vi "Main.vi"() -> ()   [LabVIEW 2021]
uses:
  Sub VIs/State Estimator/Measurements.ctl
  Sub VIs/IMU/IMU Data.ctl
  Sub VIs/Steering Motor Encoder/Steering Motor Encoder Data.ctl
  Sub VIs/GNSS/GNSS Data.ctl
  Sub VIs/State Estimator/State Estimate.ctl
  Sub VIs/Logging/Controller Data.ctl
  Sub VIs/Drive Motor/Drive Motor Data.ctl
  Sub VIs/Steering Motor/Steering Motor Data.ctl
  <vilib>/Utility/RT CPU Load.ctl
  Sub VIs/Trajectory Control/Trajectory_Control.ctl
  Sub VIs/Logging/Log Level.ctl
  <vilib>/Platform/TimedLoop/XDataNode/timing_clust.ctl
  <vilib>/Platform/TimedLoop/XDataNode/nitl_modes.ctl
  <vilib>/Platform/TimedLoop/XDataNode/wakeup.ctl
  <vilib>/platform/TimedLoop/XDataNode/XDataNode.xnode
  <vilib>/Platform/TimedLoop/XDataNode/XDNodeRunTimeDep.lvlib
  <vilib>/NI_Real-Time Target Support.lvlib
panel:
  out "XY trajectory (0 is bikeposition)":T1(graph)
  out "Y-Offset":dbl
  out "X-Offset":dbl
  out "Trajectory (Debug)":T2
  in  "Reset and Init trajectory":bool
  out "CPU loads":T3[](array[typedef]) {"ISR (%)" format="%#.2f"; "Idle (%)" format="%#.2f"; "Background (%)" format="%#.2f"; "Normal (%)" format="%#.2f"; "Above Normal (%)" format="%#.2f"; "High (%)" format="%#.2g"; "Timed Structures (%)" format="%#.2g"; "Time Critical (%)" format="%#.2g"; "Total (%)" format="%#.2g"}
  in  "Drive Motor Angular Speed (rad/s)":dbl
  out "Motor Controllers (Debug)":T4
  in  "Enable Steering Motor":bool
  out "Steering Motor Enabled":bool
  out "State Estimate (Debug)":T7 {"Y (m)" format="%#_10g"; "X (m)" format="%#_10g"}
  out "Measurements (Debug)":T8 {"GNSS Data"."Longitude (deg)" format="%#.10g"; "GNSS Data"."Latitude (deg)" format="%#.10g"; "GNSS Data"."Longitude (rad)" format="%#_10g"; "GNSS Data"."Latitude (rad)" format="%#_10g"}
  out "Abort":bool
  in  "Reset Steering Motor Encoder":bool
  in  "Stop Button":bool
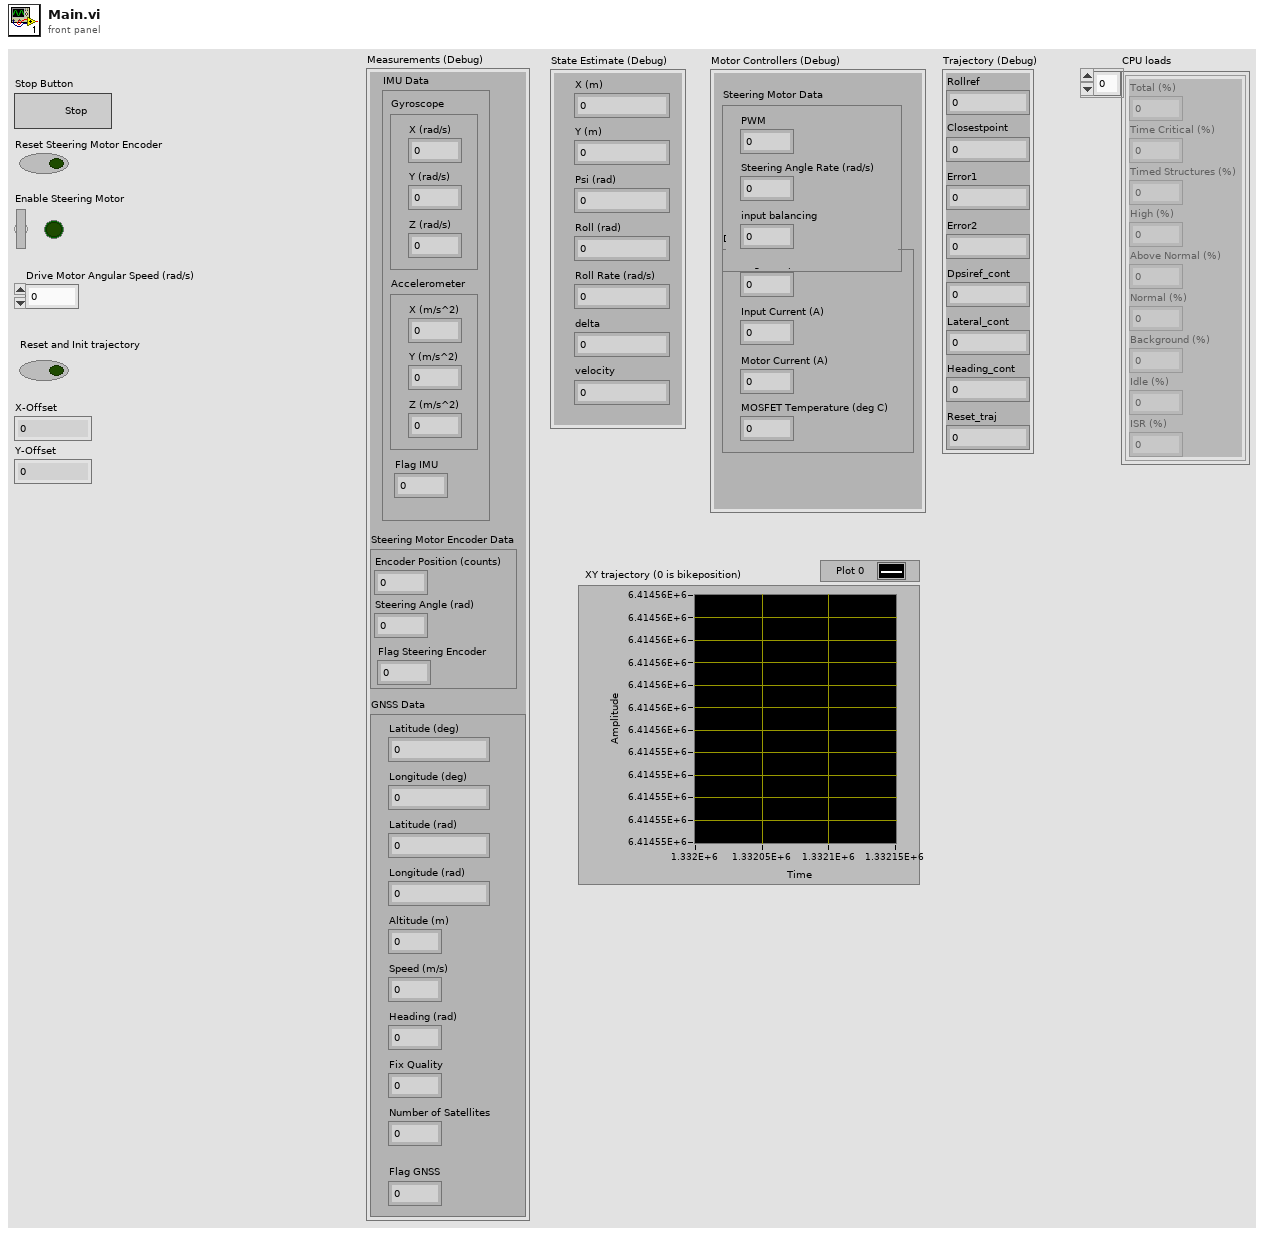
[diagram p1: front panel]
types:
  T1 = cluster{"Trajectory(X/Y/PSI)":dbl[], "Trajectory(X/Y/PSI)":dbl[]}
  T2 = typedef "Trajectory_Control.ctl" = cluster{"Rollref":dbl, "Closestpoint":dbl, "Error1":dbl, "Error2":dbl, "Dpsiref_cont":dbl, "Lateral_cont":dbl, "Heading_cont":dbl, "Reset_traj":dbl}
  T3 = typedef "NI_Real-Time Target Support.lvlib/RT CPU Load.ctl" = cluster{"Total (%)":dbl, "Time Critical (%)":dbl, "Timed Structures (%)":dbl, "High (%)":dbl, "Above Normal (%)":dbl, "Normal (%)":dbl, "Background (%)":dbl, "Idle (%)":dbl, "ISR (%)":dbl}
  T4 = typedef "Controller Data.ctl" = cluster{"Drive Motor Data":T5, "Steering Motor Data":T6}
  T5 = typedef "Drive Motor Data.ctl" = cluster{"Angular Speed (rad/s)":dbl, "Input Current (A)":dbl, "Motor Current (A)":dbl, "MOSFET Temperature (deg C)":dbl}
  T6 = typedef "Steering Motor Data.ctl" = cluster{"PWM":dbl, "Steering Angle Rate (rad/s)":dbl, "input balancing":dbl}
  T7 = typedef "State Estimate.ctl" = cluster{"X (m)":dbl, "Y (m)":dbl, "Psi (rad)":dbl, "Roll (rad)":dbl, "Roll Rate (rad/s)":dbl, "delta":dbl, "velocity":dbl}
  T8 = typedef "Measurements.ctl" = cluster{"IMU Data":T9, "Steering Motor Encoder Data":T10, "GNSS Data":T11}
  T9 = typedef "IMU Data.ctl" = cluster{"Gyroscope":cluster{"X (rad/s)":dbl, "Y (rad/s)":dbl, "Z (rad/s)":dbl}, "Accelerometer":cluster{"X (m/s^2)":dbl, "Y (m/s^2)":dbl, "Z (m/s^2)":dbl}, "Flag IMU":dbl}
  T10 = typedef "Steering Motor Encoder Data.ctl" = cluster{"Encoder Position (counts)":i32, "Steering Angle (rad)":dbl, "Flag Steering Encoder":dbl}
  T11 = typedef "GNSS Data.ctl" = cluster{"Latitude (rad)":dbl, "Longitude (rad)":dbl, "Altitude (m)":dbl, "Speed (m/s)":dbl, "Heading (rad)":dbl, "Fix Quality":i32, "Number of Satellites":i32, "Latitude (deg)":dbl, "Longitude (deg)":dbl, "Flag GNSS":dbl}
  T12 = typedef "XDNodeRunTimeDep.lvlib/timing_clust.ctl" = cluster{"Expected End [f-1]":u64, "Actual End [f-1]":u64, "Finished Late? [f-1]":bool, "Expected End [i-1]":u64, "Actual End [i-1]":u64, "Finished Late? [i-1]":bool, "Expected Start [i]":u64, "Actual Start [i]":u64, "Expected Start [f]":u64, "Actual Start [f]":u64, "Source Name":string, "Structure Name":string, "Period":i64, "Deadline":i64, "Offset":i64, "Start":i64, "Priority":i32, "Timeout":i32, "Mode":T13, "Wakeup Reason":T14, "Error":errorcluster, "Source Type":string, "Secondary Source Type":string, "Global End Time":u64, "Global Start Time":u64, "Frame Duration":u64, "Iteration Duration":u64, "Assigned CPU":i32, "I/O Scan Engine Mode":u32}
  T13 = typedef "XDNodeRunTimeDep.lvlib/nitl_modes.ctl" = enum32{"No Change", "Process missed periods, maintain original phase", "Discard missed periods, maintain original phase", "Process missed periods, ignore original phase", "Discard missed periods, ignore original phase"}
  T14 = typedef "XDNodeRunTimeDep.lvlib/wakeup.ctl" = enum32{"Normal", "Aborted", "Asynchronous wakeup", "Timing source error", "Timed loop error", "Timeout"}
  T15 = typedef "Log Level.ctl" = enum16{"Error", "Warning", "Info"}
  T16 = cluster{"B":dbl[], "A":dbl[][], "C":dbl[][], "D":dbl[], "K":dbl[][], "Trajectory(X/Y/PSI)":dbl[][], "Init":dbl[]}
  T17 = typedef "Configuration.ctl" = cluster{"Accelerometer Bias":cluster{"X (m/s)":dbl, "Y (m/s)":dbl, "Z (m/s)":dbl}, "Gyroscope Bias":cluster{"X (m/s)":dbl, "Y (m/s)":dbl, "Z (m/s)":dbl}, "Steering Motor Gear Ratio":dbl, "Steering Pully Gear Ratio":dbl, "Steering Encoder CPR":dbl, "Steering Motor Max RPM":dbl, "Wheelbase (m)":dbl, "Fork Angle (rad)":dbl, "Balancing Controller":cluster{"Kp (/s)":dbl, "Kd (1)":dbl}, "Max Allowed Steering Angle (rad)":dbl, "Task Periods":cluster{"Emergency Stop (us)":i64, "IMU (us)":i64, "Steering Motor Encoder (us)":i64, "State Estimator (us)":i64, "Balancing Controller (us)":i64, "GNSS (us)":i64, "Logging (us)":i64, "Drive Motor (us)":i64}, "Drive Motor Gear Ratio":dbl, "lr":dbl, "lf":dbl, "lambda":dbl, "k1":dbl, "k2":dbl, "e1_max":dbl, "Ad_t":dbl, "Bd_t":dbl, "C_t":dbl, "D_t":dbl, "Wheel radius":dbl}
  T18 = typedef "NI_Matrix.lvlib/RealMatrix.ctl" = dbl[][]
  T19 = typedef "IMU Handle.ctl" = cluster{"I2C address":u8}
  T20 = typedef "GNSS Handle.ctl" = cluster{"VISA Resource Name":refnum<visa-resource-name>}
  T21 = typedef "Drive Motor Handle.ctl" = cluster{"VISA Resource Name":refnum<visa-resource-name>}
  T22 = typedef "Steering Motor Handle.ctl" = cluster{"Dummy":dbl}
  T23 = typedef "Log Handle.ctl" = cluster{"Data File":refnum<file>, "Event File":refnum<file>}
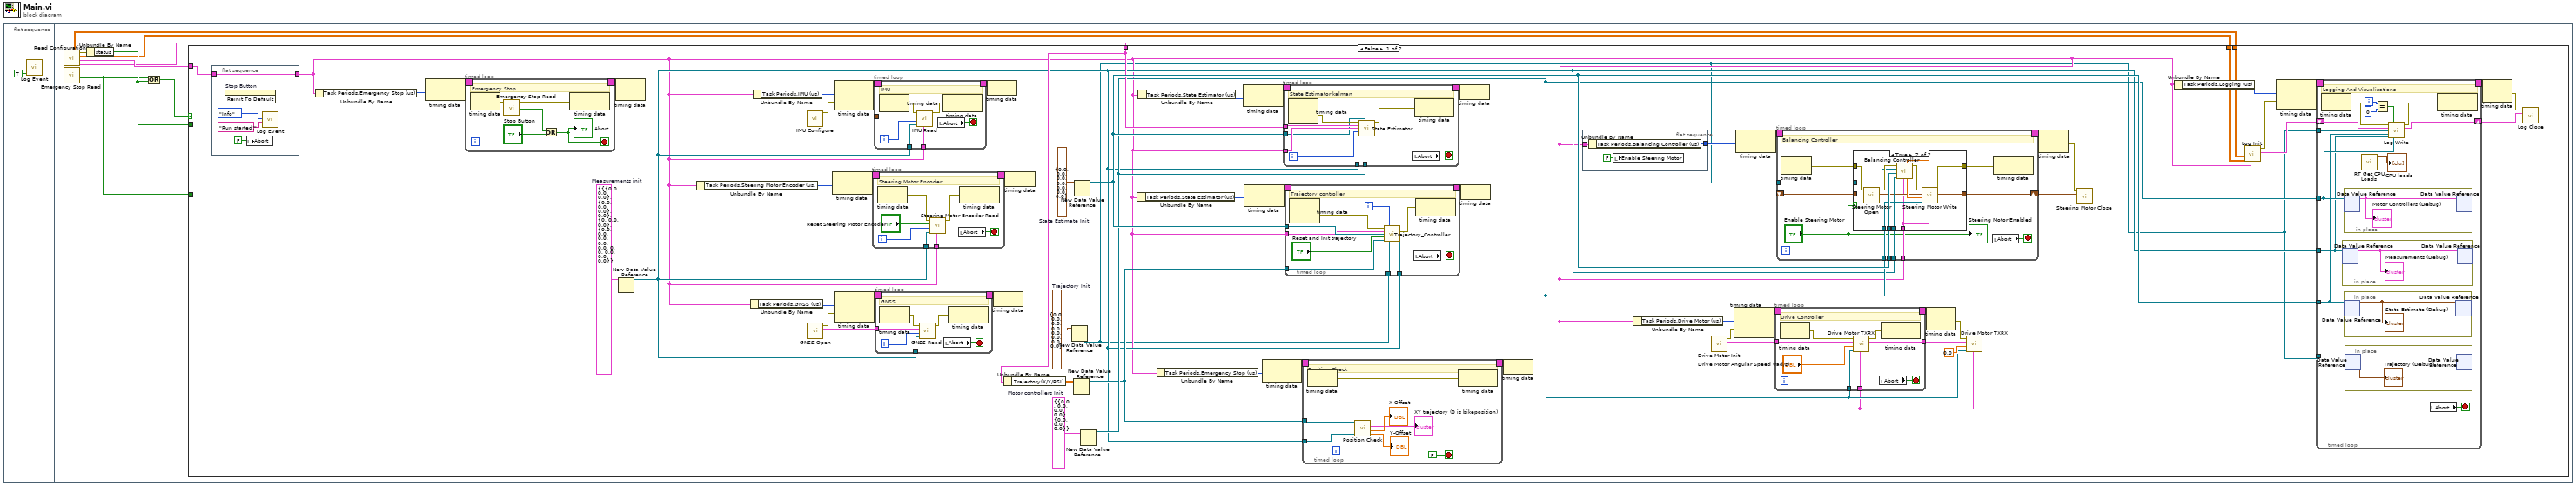
[diagram p0: block diagram]
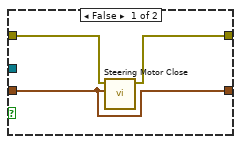
[diagram p2: hidden frame]
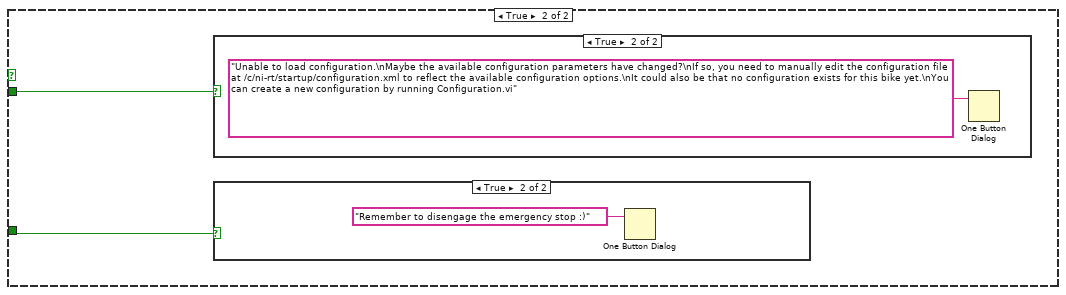
[diagram p3: hidden frame]
diagram:
  n1 = flat-sequence {
    frame #0 {
      n2 = call "Log Event.vi"("Clear Log"=TRUE) -> ()  [unwired: 10 in, 1 out]
    }
    frame #1 {
      n3 = call "Read Configuration.vi"() -> ("Matrices"=w7:T16, "Configuration"=w9:T17, "value"=w2:T18, "Error Out"=w8:errorcluster, "init trajectory 2"=w4:dbl[][])  [unwired: 7 in]
      n4 = call "Emergency Stop Read.vi"() -> ("Emergency Stop"=w5:bool)  [unwired: 10 in, 1 out]
      n5 = Unbundle By Name(w8) -> ("status"=w6:bool)
      n6 = Compound Arithmetic op=OR(w5, w6) -> (w3:bool)
      n7 = case shown="False" w3 {
        tunnel: w6 -> [_ w279]
        tunnel: w9 -> [w47 _]
        tunnel: w7 -> [w21 _]
        tunnel: w5 -> [_ w278]
        tunnel: w4 -> [w38 _]
        tunnel: w2 -> [w15 _]
        frame False {
          w23 = T2 {"Rollref"=0.0, "Closestpoint"=0.0, "Error1"=0.0, "Error2"=0.0, "Dpsiref_cont"=0.0, "Lateral_cont"=0.0, "Heading_cont"=0.0, "Reset_traj"=0.0}  # Trajectory Init
          w39 = T7 {"X (m)"=0.0, "Y (m)"=0.0, "Psi (rad)"=0.0, "Roll (rad)"=0.0, "Roll Rate (rad/s)"=0.0, "delta"=0.0, "velocity"=0.0}  # State Estimate Init
          w46 = T4 {"Drive Motor Data"={"Angular Speed (rad/s)"=0.0, "Input Current (A)"=0.0, "Motor Current (A)"=0.0, "MOSFET Temperature (deg C)"=0.0}, "Steering Motor Data"={"PWM"=0.0, "Steering Angle Rate (rad/s)"=0.0, "input balancing"=0.0}}  # Motor controllers Init
          w69 = T8 {"IMU Data"={"Gyroscope"={"X (rad/s)"=0.0, "Y (rad/s)"=0.0, "Z (rad/s)"=0.0}, "Accelerometer"={"X (m/s^2)"=0.0, "Y (m/s^2)"=0.0, "Z (m/s^2)"=0.0}, "Flag IMU"=0.0}, "Steering Motor Encoder Data"={"Encoder Position (counts)"=0, "Steering Angle (rad)"=0.0, "Flag Steering Encoder"=0.0}, "GNSS Data"={"Latitude (rad)"=0.0, "Longitude (rad)"=0.0, "Altitude (m)"=0.0, "Speed (m/s)"=0.0, "Heading (rad)"=0.0, "Fix Quality"=0, "Number of Satellites"=0, "Latitude (deg)"=0.0, "Longitude (deg)"=0.0, "Flag GNSS"=0.0}}  # Measurements init
          n8 = flat-sequence {
            tunnel: [w274] -> w11
            tunnel: w47 -> [w274]
            frame #0 {
              n9 = invoke on="Stop Button" class="Bool (strict)" method="Reinit To Default"() -> ()  [unwired: 3 in, 3 out]
              n10 = local write "Abort"(FALSE ("Abort")) -> ()
              n11 = call "Log Event.vi"("Message"="Run started!", "Log Level"=Log_Level."Info") -> ()  [unwired: 9 in, 1 out]
            }
          }
          n12 = Unbundle By Name(w11) -> ("Task Periods.Emergency Stop (us)"=w68:i64)
          n13 = node-c288(w68) -> (w67:T12)
          n14 = timed-loop {
            timing: w67 -> [_]
            timing-out: [_] -> w66
            stop <- w260 stop-if-true
            # "Emergency Stop"
            n15 = node-c288() -> (w264:errorcluster)  [unwired: 1 in]
            n16 = call "Emergency Stop Read.vi"("Error In"=w264) -> ("Emergency Stop"=w262:bool, "Error Out"=w263:errorcluster)  [unwired: 9 in]
            n17 = Or(x=w262, y="Stop Button") -> (x .or. y?=w260:bool)
            "Abort" <- w260
            n18 = node-c288(w263) -> ()  [unwired: 1 out]
          }
          n19 = node-c288(w66) -> ()  [unwired: 1 out]
          n20 = New Data Value Reference(data value=w69) -> (data value reference=w12:refnum<data-value>)  [unwired: 1 in, 1 out]
          n21 = Unbundle By Name(w11) -> ("Task Periods.Steering Motor Encoder (us)"=w52:i64)
          n22 = Unbundle By Name(w11) -> ("Task Periods.GNSS (us)"=w49:i64)
          n23 = Unbundle By Name(w11) -> ("Task Periods.IMU (us)"=w53:i64)
          n24 = call "IMU Configure.vi"() -> ("IMU Handle"=w54:T19, "Error Out"=w55:errorcluster)  [unwired: 10 in]
          n25 = call "GNSS Open.vi"() -> ("GNSS Handle"=w50:T20, "Error Out"=w51:errorcluster)  [unwired: 10 in]
          n26 = node-c288(w52) -> (w59:T12)
          n27 = node-c288(w53, w55) -> (w61:T12)
          n28 = node-c288(w49, w51) -> (w57:T12)
          n29 = timed-loop {
            timing: w59 -> [_]
            timing-out: [_] -> w58
            tunnel: w12 -> [w189]
            tunnel: w11 -> [w187]
            i -> [w188]
            stop <- w190 stop-if-true
            # "Steering Motor Encoder"
            n30 = node-c288() -> (w193:errorcluster)  [unwired: 1 in]
            n31 = call "Steering Motor Encoder Read.vi"("Configuration"=w187, "Measurement In"=w189, "Flag Steering Encoder"=w188, "Reset Counter"="Reset Steering Motor Encoder", "Error In"=w193) -> ("Error Out"=w192:errorcluster)  [unwired: 4 in, 2 out]
            n32 = local read "Abort"() -> (w190:bool)
            n33 = node-c288(w192) -> ()  [unwired: 1 out]
          }
          n34 = timed-loop {
            timing: w61 -> [_]
            timing-out: [_] -> w60
            tunnel: w54 -> [w207]
            tunnel: w12 -> [w205]
            tunnel: w11 -> [w204]
            i -> [w203]
            stop <- w206 stop-if-true
            # "IMU"
            n35 = node-c288() -> (w209:errorcluster)  [unwired: 1 in]
            n36 = call "IMU Read.vi"("Configuration"=w204, "Measurement In"=w205, "Flag IMU"=w203, "IMU Handle"=w207, "Error In"=w209) -> ("Error Out"=w208:errorcluster)  [unwired: 4 in, 2 out]
            n37 = local read "Abort"() -> (w206:bool)
            n38 = node-c288(w208) -> ()  [unwired: 1 out]
          }
          n39 = timed-loop {
            timing: w57 -> [_]
            timing-out: [_] -> w56
            tunnel: w50 -> [w176]
            tunnel: w12 -> [w172]
            i -> [w171]
            stop <- w173 stop-if-true
            # "GNSS"
            n40 = node-c288() -> (w175:errorcluster)  [unwired: 1 in]
            n41 = call "GNSS Read.vi"("Measurement In"=w172, "Flag GNSS"=w171, "GNSS Handle"=w176, "Error In"=w175) -> ("Error Out"=w174:errorcluster)  [unwired: 5 in, 2 out]
            n42 = local read "Abort"() -> (w173:bool)
            n43 = node-c288(w174) -> ()  [unwired: 1 out]
          }
          n44 = node-c288(w60) -> ()
          n45 = node-c288(w56) -> ()
          n46 = Unbundle By Name(w21) -> ("Trajectory(X/Y/PSI)"=w20:dbl[][])
          n47 = node-c288(w58) -> ()
          n48 = New Data Value Reference(data value=w23) -> (data value reference=w10:refnum<data-value>)  [unwired: 1 in, 1 out]
          n49 = New Data Value Reference(data value=w20) -> (data value reference=w13:refnum<data-value>)  [unwired: 1 in, 1 out]
          n50 = New Data Value Reference(data value=w39) -> (data value reference=w22:refnum<data-value>)  [unwired: 1 in, 1 out]
          n51 = New Data Value Reference(data value=w46) -> (data value reference=w14:refnum<data-value>)  [unwired: 1 in, 1 out]
          n52 = Unbundle By Name(w11) -> ("Task Periods.State Estimator (us)"=w24:i64)
          n53 = Unbundle By Name(w11) -> ("Task Periods.State Estimator (us)"=w27:i64)
          n54 = Unbundle By Name(w11) -> ("Task Periods.Emergency Stop (us)"=w16:i64)
          n55 = node-c288(w27) -> (w29:T12)
          n56 = node-c288(w24) -> (w26:T12)
          n57 = node-c288(w16) -> (w18:T12)
          n58 = timed-loop {
            timing: w29 -> [_]
            timing-out: [_] -> w28
            tunnel: w12 -> [w107]
            tunnel: w21 -> [w110]
            tunnel: w14 -> [w106]
            tunnel: w22 -> [w105]
            tunnel: w11 -> [w109]
            i -> [w108]
            stop <- w113 stop-if-true
            # "State Estimator kalman"
            n59 = node-c288() -> (w112:errorcluster)  [unwired: 1 in, 1 out]
            n60 = call "State Estimator.vi"("Error In"=w112, "State Estimate In"=w105, "Matrices"=w110, "Configuration"=w109, "Iteration"=w108, "Measurement In"=w107, "Balancing controller In"=w106) -> ("Error out"=w111:errorcluster)  [unwired: 7 in, 1 out]
            n61 = local read "Abort"() -> (w113:bool)
            n62 = node-c288(w111) -> ()  [unwired: 1 out]
          }
          n63 = timed-loop {
            timing: w26 -> [_]
            timing-out: [_] -> w25
            tunnel: w22 -> [w94]
            tunnel: w11 -> [w91]
            tunnel: w12 -> [w89]
            tunnel: w13 -> [w88]
            tunnel: w10 -> [w86]
            i -> [w90]
            stop <- w95 stop-if-true
            # "Trajectory controller"
            n64 = node-c288() -> (w92:errorcluster)  [unwired: 1 in, 1 out]
            n65 = call "Trajectory_Controller.vi"("Error In"=w92, "reset"=w90, "Configuration"=w91, "State Estimate In"=w94, "Reset and Init trajectory"="Reset and Init trajectory", "RefTraj in"=w88, "Trajectory In"=w86, "Measurement In"=w89) -> ("Error out"=w93:errorcluster)  [unwired: 5 in, 2 out]
            n66 = local read "Abort"() -> (w95:bool)
            n67 = node-c288(w93) -> ()  [unwired: 1 out]
          }
          n68 = timed-loop {
            timing: w18 -> [_]
            timing-out: [_] -> w17
            tunnel: w13 -> [w74]
            tunnel: w12 -> [w73]
            stop <- FALSE stop-if-true
            # "Position Check"
            n69 = node-c288() -> (w76:errorcluster)  [unwired: 1 in]
            n70 = call "Position Check.vi"("data value reference 2"=w73, "data value reference"=w74) -> ("Y-Offset"=→"Y-Offset":dbl, "X-Offset"=→"X-Offset":dbl, "XY Graph"=→"XY trajectory (0 is bikeposition)":T1)  [unwired: 7 in]
            n71 = node-c288(w76) -> ()  [unwired: 1 out]
          }
          n72 = node-c288(w28) -> ()
          n73 = node-c288(w25) -> ()
          n74 = node-c288(w17) -> ()
          n75 = flat-sequence {
            tunnel: [w221] -> w48
            tunnel: w11 -> [w220]
            frame #0 {
              n76 = Unbundle By Name(w220) -> ("Task Periods.Balancing Controller (us)"=w221:i64)
              n77 = local write "Enable Steering Motor"(FALSE ("Enable Steering Motor")) -> ()
            }
          }
          n78 = Unbundle By Name(w11) -> ("Task Periods.Drive Motor (us)"=w35:i64)
          n79 = call "Drive Motor Init.vi"() -> ("Drive Motor Handle"=w34:T21, "Error Out"=w33:errorcluster)  [unwired: 10 in]
          n80 = node-c288(w35, w33) -> (w37:T12)
          n81 = node-c288(w48) -> (w65:T12)
          n82 = timed-loop {
            timing: w37 -> [_]
            timing-out: [_] -> w36
            tunnel: w34 -> [w128]
            tunnel: w11 -> [w127]
            tunnel: w14 -> [w126]
            tunnel: [w129] -> w30
            stop <- w130 stop-if-true
            # "Drive Controller"
            n83 = node-c288() -> (w124:errorcluster)  [unwired: 1 in]
            n84 = call "Drive Motor TXRX.vi"("Configuration"=w127, "Controller Data In"=w126, "Angular Speed (rad/s)"="Drive Motor Angular Speed (rad/s)", "Drive Motor Handle In"=w128, "Error In"=w124) -> ("Drive Motor Handle Out"=w129:T21, "Error Out"=w123:errorcluster)  [unwired: 3 in, 2 out]
            n85 = local read "Abort"() -> (w130:bool)
            n86 = node-c288(w123) -> ()  [unwired: 1 out]
          }
          n87 = timed-loop {
            timing: w65 -> [_]
            timing-out: [_] -> w64
            tunnel: w22 -> [w229]
            tunnel: w12 -> [w228]
            shift-right: [w230] -> w63
            shift-left: _ -> [w227]
            tunnel: w11 -> [w226]
            tunnel: w14 -> [w225]
            tunnel: w10 -> [w223]
            stop <- w233 stop-if-true
            # "Balancing Controller"
            n88 = node-c288() -> (w232:errorcluster)  [unwired: 1 in]
            n89 = case shown="True" "Enable Steering Motor" {
              tunnel: w232 -> [w236 w243]
              tunnel: [w235 w248] -> w231
              tunnel: [w234 w247] -> w230
              tunnel: w229 -> [_ w245]
              tunnel: w228 -> [_ w244]
              tunnel: w227 -> [w234 _]
              tunnel: w226 -> [_ w239]
              tunnel: w225 -> [_ w240]
              tunnel: w223 -> [_ w238]
              frame False {
                n90 = call "Steering Motor Close.vi"("Steering Motor Handle"=w234, "Error In"=w236) -> ("Error Out"=w235:errorcluster)  [unwired: 9 in]
              }
              frame True {
                n91 = call "Steering Motor Open.vi"("Error In"=w243) -> ("Steering Motor Handle"=w241:T22, "Error Out"=w242:errorcluster)  [unwired: 9 in]
                n92 = call "Balancing Controller.vi"("Configuration"=w239, "Measurement In"=w244, "State Estimate In"=w245, "Trajectory In"=w238, "Error In"=w242) -> ("Error Out"=w249:errorcluster, "Steering Angle Rate (rad/s)"=w246:dbl, "Input balancing"=w237:dbl)  [unwired: 2 in, 2 out]
                n93 = call "Steering Motor Write.vi"("Configuration"=w239, "Numeric"=w237, "Controller Data In"=w240, "Steering Angle Rate (rad/s)"=w246, "Steering Motor Handle In"=w241, "Error In"=w249) -> ("Steering Motor Handle Out"=w247:T22, "Error Out"=w248:errorcluster)  [unwired: 2 in, 2 out]
              }
            }
            n94 = local read "Abort"() -> (w233:bool)
            n95 = node-c288(w231) -> ()  [unwired: 1 out]
            "Steering Motor Enabled" <- "Enable Steering Motor"
          }
          n96 = node-c288(w36) -> (w32:errorcluster)
          n97 = call "Drive Motor TXRX.vi"("Configuration"=w11, "Controller Data In"=w14, "Angular Speed (rad/s)"=0.0, "Drive Motor Handle In"=w30, "Error In"=w32) -> ()  [unwired: 3 in, 4 out]
          n98 = node-c288(w64) -> (w62:errorcluster)
          n99 = call "Steering Motor Close.vi"("Steering Motor Handle"=w63, "Error In"=w62) -> ()  [unwired: 9 in, 1 out]
          n100 = Unbundle By Name(w11) -> ("Task Periods.Logging (us)"=w43:i64)
          n101 = call "Log Init.vi"("Configuration"=w11, "Matrices"=w15, "Trajectory"=w38) -> ("Log Handle"=w40:T23, "Error Out"=w42:errorcluster)  [unwired: 7 in]
          n102 = node-c288(w43, w42) -> (w45:T12)
          n103 = timed-loop {
            timing: w45 -> [_]
            timing-out: [_] -> w44
            tunnel: w12 -> [w142]
            tunnel: w22 -> [w147]
            shift-right: [w149] -> w19
            shift-left: w40 -> [w148]
            tunnel: w14 -> [w146]
            tunnel: w10 -> [w145]
            tunnel: w10 -> [w143]
            i -> [w154]
            stop <- w155 stop-if-true
            # "Logging And Visualisations"
            n104 = node-c288() -> (w151:errorcluster)  [unwired: 1 in]
            n105 = in-place {
              n106 = in-place-dvr #1(w142) -> (w159:T8)  [unwired: 1 out]
              "Measurements (Debug)" <- w159
              n107 = in-place-dvr #1(w159) -> ()  [unwired: 2 out]
            }
            n108 = in-place {
              n109 = in-place-dvr #2(w146) -> (w157:T4)  [unwired: 1 out]
              "Motor Controllers (Debug)" <- w157
              n110 = in-place-dvr #2(w157) -> ()  [unwired: 2 out]
            }
            n111 = in-place {
              n112 = in-place-dvr #3(w147) -> (w158:T7)  [unwired: 1 out]
              "State Estimate (Debug)" <- w158
              n113 = in-place-dvr #3(w158) -> ()  [unwired: 2 out]
            }
            n114 = in-place {
              n115 = in-place-dvr #4(w143) -> (w156:T2)  [unwired: 1 out]
              "Trajectory (Debug)" <- w156
              n116 = in-place-dvr #4(w156) -> ()  [unwired: 2 out]
            }
            n117 = call <vilib>:"RT Get CPU Loads.vi"() -> ("CPU loads"=→"CPU loads":T3[])  [unwired: 10 in, 1 out]
            n118 = Equal?(x=w154, y=0) -> (x = y?=w152:bool)
            n119 = call "Log Write.vi"("Error In"=w151, "Write Header"=w152, "Log Handle In"=w148, "Trajectory In"=w145, "State Estimate In"=w147, "Measurement In"=w142, "Controller Data In"=w146) -> ("Error Out"=w150:errorcluster, "Log Handle Out"=w149:T23)  [unwired: 2 in, 5 out]
            n120 = local read "Abort"() -> (w155:bool)
            n121 = node-c288(w150) -> ()  [unwired: 1 out]
          }
          n122 = node-c288(w44) -> (w41:errorcluster)
          n123 = call "Log Close.vi"("Log Handle In"=w19, "Error In"=w41) -> ()  [unwired: 9 in, 1 out]
        }
        frame True {
          n124 = case shown="True" w279 {
            frame False {
            }
            frame True {
              n125 = One Button Dialog(message="Unable to load configuration.\nMaybe the available configuration parameters have changed?\nIf so, you need to manually edit the configuration file at /c/ni-rt/startup/configuration.xml to reflect the available configuration options.\nIt could also be that no configuration exists for this bike yet.\nYou can create a new configuration by running Configuration.vi") -> ()  [unwired: 1 in, 1 out]
            }
          }
          n126 = case shown="True" w278 {
            frame False {
            }
            frame True {
              n127 = One Button Dialog(message="Remember to disengage the emergency stop :)") -> ()  [unwired: 1 in, 1 out]
            }
          }
        }
      }
    }
  }
